vi "oa_Get Tach Points and Timebase Data from Resampled Data.vi"(0 "resampled signal in":cluster{"r0":dbl, "dr":dbl, "Y":dbl[]}[](array[cluster]) {"r0" format="%.2p"; "dr" format="%.2p"; "Y" format="%.2f"}, 1 "tach duty":i32=1, 9 "interpolated pulse positions [s]":dbl[](array[numeric]) format="%.2f", 11 "error in":errorcluster, 12 "trigger pulse direction":u16(ring)=1 items=["positive going", "negative going"]) -> (4 "X axis":cluster{dbl[], dbl[]}[](array[cluster]) {"?" format="%.2f"; "?" format="%.2f"}, 6 "Y axis":cluster{dbl[], dbl[]}[](array[cluster]) {"?" format="%.2f"; "?" format="%.2f"}, 15 "error out":errorcluster)   [LabVIEW 2017]
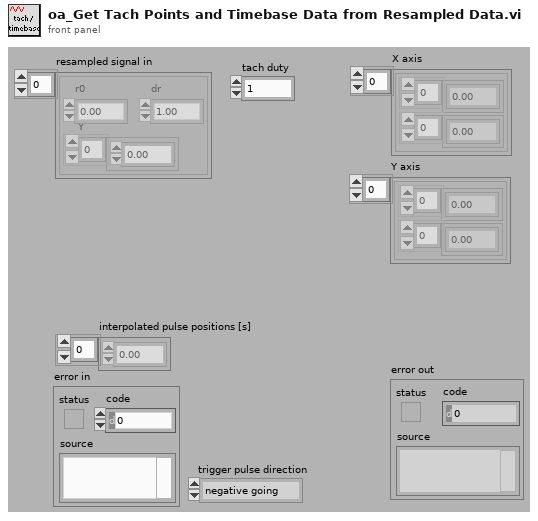
[diagram p1: front panel]
types:
  T1 = cluster{"interpolated pulse positions [s]":dbl[], "Y":dbl[]}
  T2 = cluster{"interpolated pulse positions [s]":dbl[], "Y":dbl[]}[]
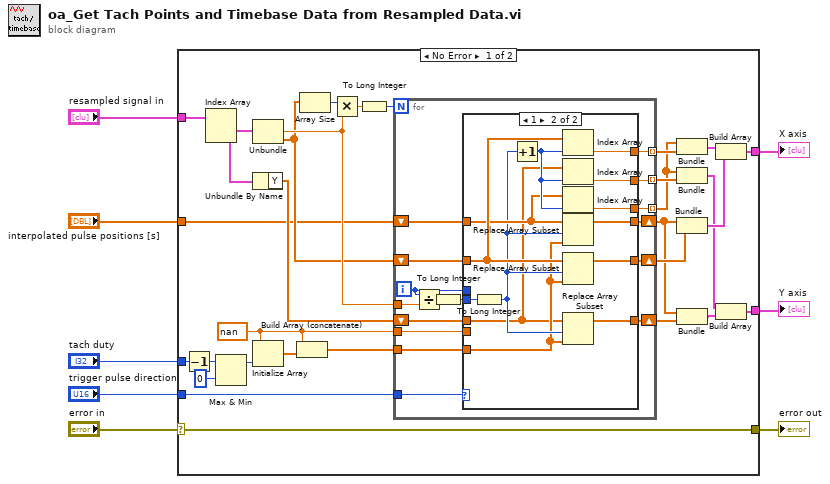
[diagram p0: block diagram]
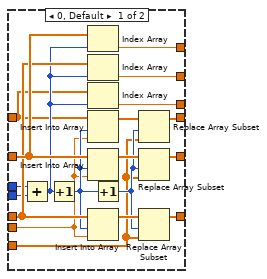
[diagram p2: hidden frame]
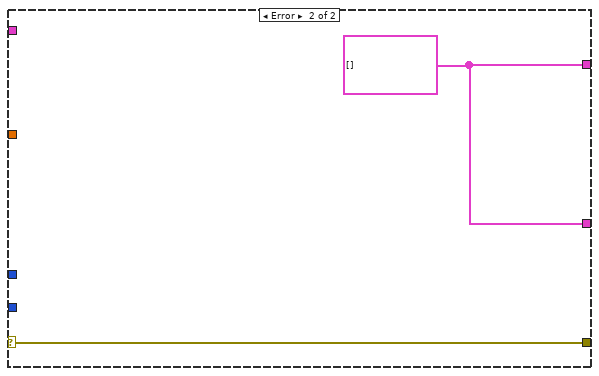
[diagram p3: hidden frame]
diagram:
  n1 = case shown="No Error" "error in" {
    selector: "error in" -> [w36 w89]
    tunnel: [w36 w89] -> w7
    tunnel: "resampled signal in" -> [w39 _]
    tunnel: [w9 w88] -> w2
    tunnel: [w12 w88] -> w3
    tunnel: "tach duty" -> [w32 _]
    tunnel: "trigger pulse direction" -> [w24 _]
    tunnel: "interpolated pulse positions [s]" -> [w21 _]
    frame No Error {
      w27 = nan ("element")
      n2 = Decrement(x=w32) -> (x-1=w31:i32)
      n3 = Index Array(array=w39) -> (element #1=w38:cluster{"r0":dbl, "dr":dbl, "Y":dbl[]}, element #2=w37:cluster{"r0":dbl, "dr":dbl, "Y":dbl[]})  [unwired: 2 in]
      n4 = Max & Min(x=w31, y=0) -> (max(x,y)=w29:i32)  [unwired: 1 out]
      n5 = Unbundle(w38) -> ("dr"=w25:dbl, "Y"=w23:dbl[])  [unwired: 1 out]
      n6 = Unbundle By Name(w37) -> ("Y"=w22:dbl[])
      n7 = Initialize Array(w27, w29) -> (w28:dbl[])
      n8 = Build Array (concatenate)(w27, w28) -> (w26:dbl[])
      n9 = Array Size(array=w23) -> (size(s)=w35:i32)
      n10 = Multiply(x=w35, y=w25) -> (x*y=w34:dbl)
      n11 = To Long Integer(number=w34) -> (32bit integer=w33:i32)
      n12 = for {
        N: w33 -> [_]
        shift-right: [w54] -> w17
        shift-left: w23 -> [w55]
        shift-right: [w52] -> w16
        shift-left: w22 -> [w53]
        tunnel: w24 -> [w51]
        tunnel: w27 -> [w50]
        tunnel: w26 -> [w49]
        tunnel: w25 -> [w48]
        tunnel: [w45] -> w20 mode=indexing
        tunnel: [w44] -> w19 mode=indexing
        shift-right: [w40] -> w15
        shift-left: w21 -> [w42]
        tunnel: [w41] -> w18 mode=indexing
        i -> [w47]
        n13 = Divide(x=w47, y=w48) -> (x/y=w46:dbl)
        n14 = To Long Integer(number=w46) -> (32bit integer=w43:i32)
        n15 = case shown="1" w51 {
          tunnel: w55 -> [w69 w84]
          tunnel: [w73 w87] -> w54
          tunnel: w53 -> [w67 w75]
          tunnel: w43 -> [w65 w86]
          tunnel: [w71 w85] -> w52
          tunnel: w50 -> [w60 _]
          tunnel: w49 -> [w57 w76]
          tunnel: w47 -> [w66 _]
          tunnel: [w70 w83] -> w45
          tunnel: [w68 w82] -> w44
          tunnel: w42 -> [w62 w79]
          tunnel: [w63 w80] -> w41
          tunnel: [w56 w78] -> w40
          frame 0, Default {
            n16 = Add(x=w66, y=w65) -> (x+y=w64:i32)
            n17 = Increment(x=w64) -> (x+1=w61:i32)
            n18 = Index Array(array=w69, index=w64) -> (element=w70:dbl)
            n19 = Index Array(array=w67, index=w64) -> (element=w68:dbl)
            n20 = Index Array(array=w62, index=w64) -> (element=w63:dbl)
            n21 = Insert Into Array(array=w62, index=w61, new element=w60) -> (w59:dbl[])
            n22 = Insert Into Array(array=w69, index=w61, new element=w60) -> (w74:dbl[])
            n23 = Insert Into Array(array=w67, index=w61, new element=w60) -> (w72:dbl[])
            n24 = Increment(x=w61) -> (x+1=w58:i32)
            n25 = Replace Array Subset(array=w59, new element=w57, index=w58) -> (w56:dbl[])
            n26 = Replace Array Subset(array=w74, new element=w57, index=w58) -> (w73:dbl[])
            n27 = Replace Array Subset(array=w72, new element=w57, index=w58) -> (w71:dbl[])
          }
          frame 1 {
            n28 = To Long Integer(number=w86) -> (32bit integer=w77:i32)
            n29 = Increment(x=w77) -> (x+1=w81:i32)
            n30 = Index Array(array=w84, index=w81) -> (element=w83:dbl)
            n31 = Index Array(array=w75, index=w81) -> (element=w82:dbl)
            n32 = Index Array(array=w79, index=w81) -> (element=w80:dbl)
            n33 = Replace Array Subset(array=w79, new element=w76, index=w77) -> (w78:dbl[])
            n34 = Replace Array Subset(array=w84, new element=w76, index=w77) -> (w87:dbl[])
            n35 = Replace Array Subset(array=w75, new element=w76, index=w77) -> (w85:dbl[])
          }
        }
      }
      n36 = Bundle(w18, w20) -> (w14:cluster{dbl[], dbl[]})  [unwired: 1 in]
      n37 = Bundle(w18, w19) -> (w10:cluster{dbl[], dbl[]})  [unwired: 1 in]
      n38 = Bundle("interpolated pulse positions [s]"=w15, "Y"=w17) -> (w13:T1)  [unwired: 1 in]
      n39 = Bundle("interpolated pulse positions [s]"=w15, "Y"=w16) -> (w11:T1)  [unwired: 1 in]
      n40 = Build Array(w14, w13) -> (w12:T2)
      n41 = Build Array(w10, w11) -> (w9:T2)
    }
    frame Error {
      w88 = cluster{dbl[], dbl[]}[] []
    }
  }
  "error out" <- w7
  "X axis" <- w3
  "Y axis" <- w2
